vi "Do.vi"(8 "error in (no error)":errorcluster, 10 "Actor in":refnum<class "Actor.lvclass">, 11 "StartMeasurement Msg":refnum<class "StartMeasurement Msg.lvclass">) -> (0 "error out":errorcluster, 2 "Actor out":refnum<class "Actor.lvclass">)   [LabVIEW 2023, in "Multiharp.lvlib" / "StartMeasurement Msg.lvclass"]
doc: "This VI delivers the message to the actor by calling the appropriate method(s) on the actor."
uses:
  StartMeasurement Msg.lvclass
  StartMeasurement Msg.lvclass/StartMeasurement Msg.ctl
  9310f1bf-65b7-4236-a38b-723b0abf1b68.vi
  Multiharp/Multiharp.lvclass
  <vilib>/ActorFramework/Actor/Actor.lvclass
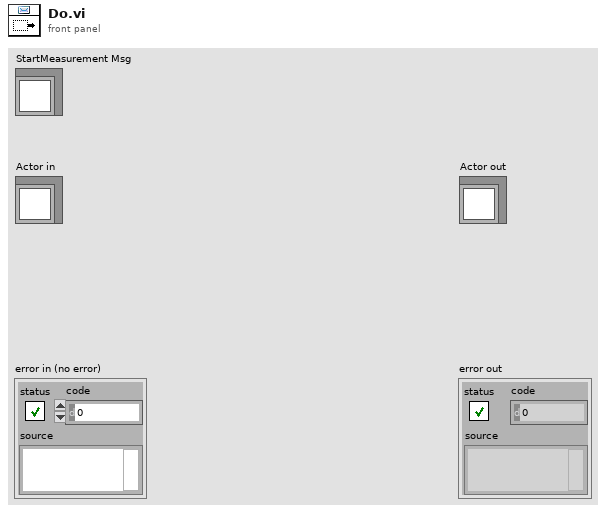
[diagram p1: front panel]
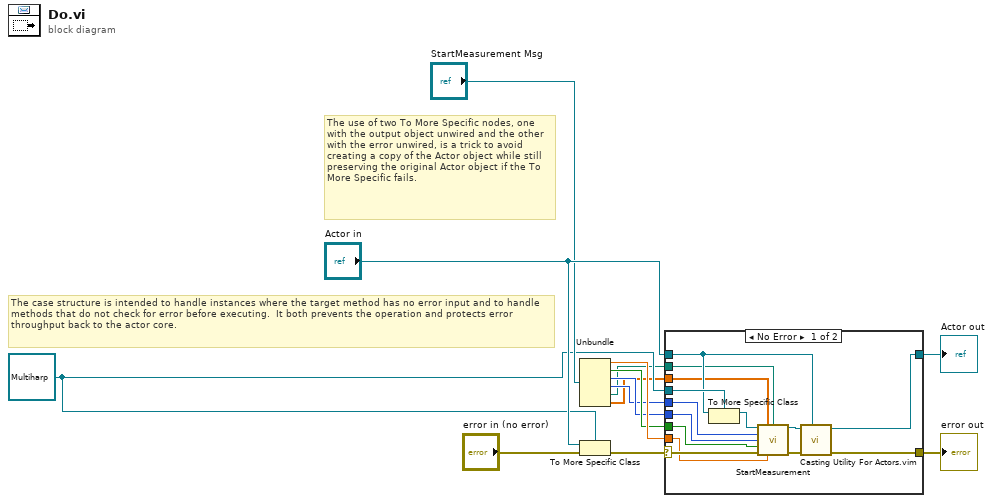
[diagram p0: block diagram]
diagram:
  w8 = refnum<class "Multiharp.lvclass"> refnum ("Actor in")
  # "The use of two To More Specific nodes, one with the output object unwired and the other with the error unwired, is a trick to avoid creating a copy of the Actor object while still preserving the original Actor object if the To More Specific fails."
  # "The case structure is intended to handle instances where the target method has no error input and to handle methods that do not check for error before executing.  It both prevents the operation and protects error throughput back to the actor core."
  n1 = Unbundle("StartMeasurement Msg") -> (w6:dbl, w5:bool, w4:i32, w3:i32, w2:path, w1:dbl[])
  n2 = To More Specific Class(target class=w8, reference="Actor in", error in="error in (no error)") -> (error out=w7:errorcluster)  [unwired: 1 out]
  n3 = case shown="No Error" w7 {
    selector: w7 -> [w27 w29]
    tunnel: [w21 w29] -> w13
    tunnel: [w22 w28] -> w12
    tunnel: "Actor in" -> [w24 w28]
    tunnel: w8 -> [w25 _]
    tunnel: w6 -> [w19 _]
    tunnel: w5 -> [w18 _]
    tunnel: w4 -> [w17 _]
    tunnel: w3 -> [w16 _]
    tunnel: w2 -> [w15 _]
    tunnel: w1 -> [w14 _]
    frame No Error {
      n4 = To More Specific Class(target class=w25, reference=w24) -> (specific class reference=w26:refnum<class "Multiharp.lvclass">)  [unwired: 1 in, 1 out]
      n5 = call-dynamic "StartMeasurement.vi"("Multiharp in"=w26, "Coincidence Delays"=w14, "Path"=w15, "tacq"=w16, "Max Triggers"=w17, "Scanning"=w18, "error in (no error)"=w27, "Coincidence Window"=w19) -> ("Multiharp out"=w23:refnum<class "Multiharp.lvclass">, "error out"=w20:errorcluster)  [unwired: 6 in]
      n6 = call "Casting Utility For Actors.vim"("type"=w24, "error in (no error)"=w20, "Actor in"=w23) -> ("error out"=w21:errorcluster, "Actor out"=w22:refnum<class "Actor.lvclass">)  [unwired: 7 in]
    }
    frame Error {
      # "If type check fails, pass the original object out again."
    }
  }
  "error out" <- w13
  "Actor out" <- w12
